vi "GraphSetting ScaleY (Wave2).vi"(6 "コマンド":T1, 8 "error in (no error)":errorcluster caption="エラー入力（エラーなし）", 9 "アクティブスケールY":u16, 10 "スケール(in)":T2, 11 "波形グラフ(Wave)ref(in)":refnum<vi>) -> (0 "error out":errorcluster caption="エラー出力", 2 "スケール(out)":T2)   [LabVIEW 2014]
uses:
  GraphSetting Scale.ctl
  TypeDef/GraphSetting DisplayFormatType.ctl
  TypeDef/GraphSetting Command.ctl
panel:
  # "スケールのスタイルとカラー"
  # "スケール係数"
  # "スケールのスタイルとカラー"
  # "スケールのスタイルとカラー"
  # "スケール係数"
  # "スケールのスタイルとカラー"
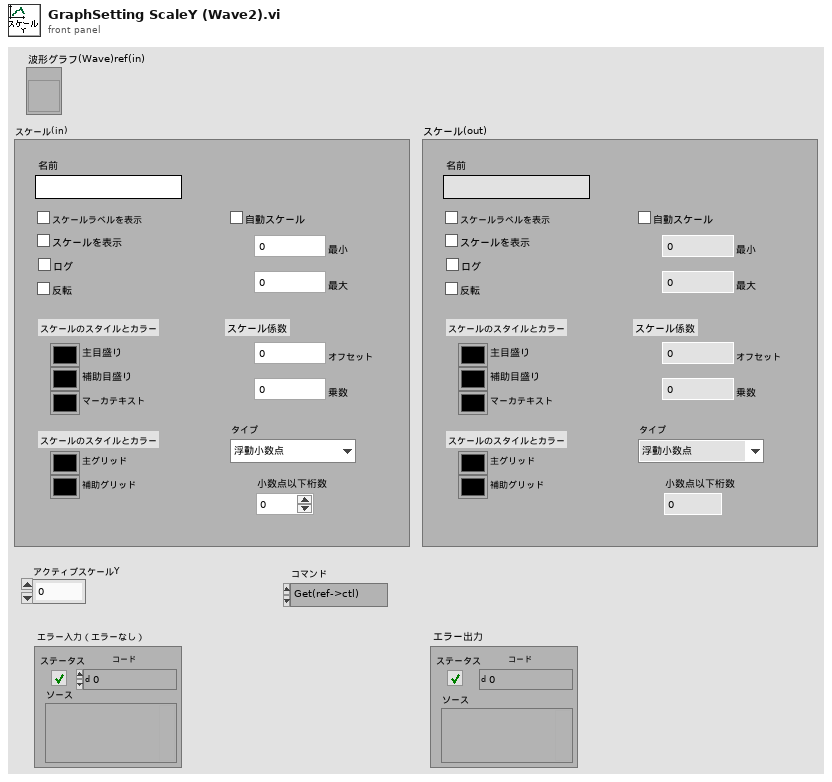
[diagram p1: front panel]
types:
  T1 = typedef "GraphSetting Command.ctl" = enum16{"Get(ref->ctl)", "Set(ctl->ref)"}
  T2 = typedef "GraphSetting Scale.ctl" = cluster{"名前":string, "スケールラベルを表示":bool, "スケールを表示":bool, "ログ":bool, "反転":bool, "自動スケール":bool, "最小":dbl, "最大":dbl, "オフセット":dbl, "乗数":dbl, "主目盛り":u32, "補助目盛り":u32, "マーカテキスト":u32, "主グリッド":u32, "補助グリッド":u32, "タイプ":T3, "小数点以下桁数":u8}
  T3 = typedef "GraphSetting DisplayFormatType.ctl" = enum8{"浮動小数点", "科学", "工学", "バイナリ", "８進数", "１６進数", "相対時間", "時間と日時", "SI"}
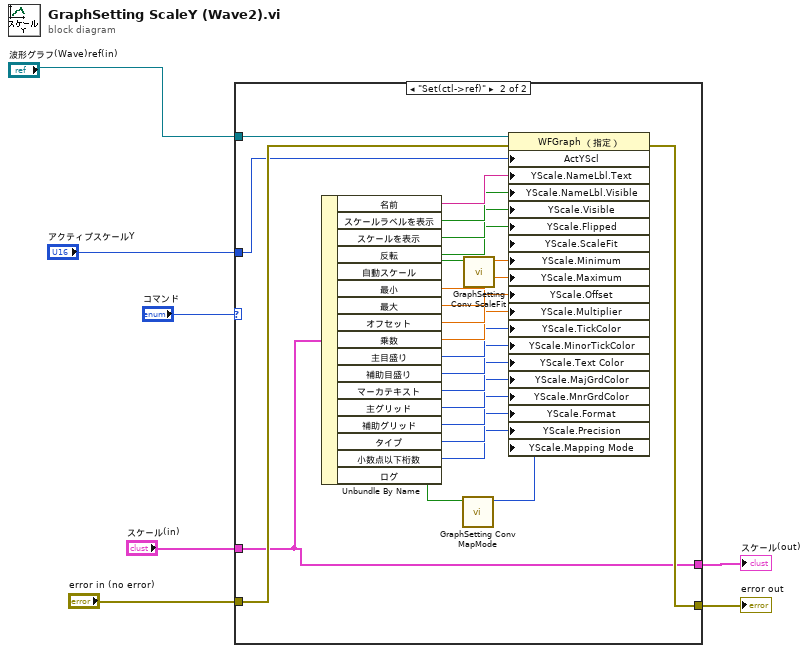
[diagram p0: block diagram]
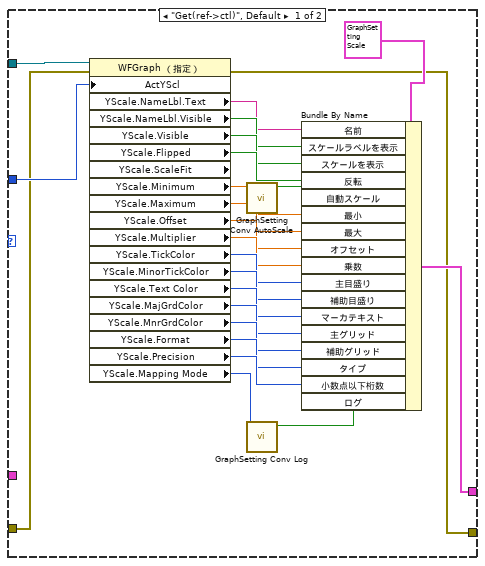
[diagram p2: hidden frame]
diagram:
  n1 = case shown="\"Set(ctl->ref)\"" "コマンド" {
    tunnel: "アクティブスケールY" -> [w16 w52]
    tunnel: "波形グラフ(Wave)ref(in)" -> [w15 w56]
    tunnel: [w14 w53] -> w6
    tunnel: [w13 w54] -> w4
    tunnel: "error in (no error)" -> [w12 w55]
    tunnel: "スケール(in)" -> [_ w53]
    frame "Get(ref->ctl)", Default {
      n2 = property class="WFGraph （指定）"(reference=w15, error in=w12, "ActYScl"=w16) -> (error out=w13:errorcluster, "YScale.NameLbl.Text"=w17:string, "YScale.NameLbl.Visible"=w18:bool, "YScale.Visible"=w19:bool, "YScale.Flipped"=w20:bool, "YScale.ScaleFit"=w11:u8, "YScale.Minimum"=w21:dbl, "YScale.Maximum"=w22:dbl, "YScale.Offset"=w23:dbl, "YScale.Multiplier"=w24:dbl, "YScale.TickColor"=w25:u32, "YScale.MinorTickColor"=w26:u32, "YScale.Text Color"=w27:u32, "YScale.MajGrdColor"=w28:u32, "YScale.MnrGrdColor"=w29:u32, "YScale.Format"=w30:u8, "YScale.Precision"=w31:u8, "YScale.Mapping Mode"=w9:u8)  [unwired: 1 out]
      n3 = call "GraphSetting Conv AutoScale.vi"("XScale.ScaleFit"=w11) -> ("自動スケール?"=w10:bool)  [unwired: 10 in]
      n4 = call "GraphSetting Conv Log.vi"("XScale.Mapping Mode"=w9) -> ("ログ?"=w8:bool)  [unwired: 10 in]
      n5 = Bundle By Name(cluster=T2 {"名前"="", "スケールラベルを表示"=FALSE, "スケールを表示"=FALSE, "ログ"=FALSE, "反転"=FALSE, "自動スケール"=FALSE, "最小"=0.0, "最大"=0.0, "オフセット"=0.0, "乗数"=0.0, "主目盛り"=0, "補助目盛り"=0, "マーカテキスト"=0, "主グリッド"=0, "補助グリッド"=0, "タイプ"=enum."浮動小数点", "小数点以下桁数"=0} ("スケール"), "名前"=w17, "スケールラベルを表示"=w18, "スケールを表示"=w19, "反転"=w20, "自動スケール"=w10, "最小"=w21, "最大"=w22, "オフセット"=w23, "乗数"=w24, "主目盛り"=w25, "補助目盛り"=w26, "マーカテキスト"=w27, "主グリッド"=w28, "補助グリッド"=w29, "タイプ"=w30, "小数点以下桁数"=w31, "ログ"=w8) -> (w14:T2)
    }
    frame "Set(ctl->ref)" {
      n6 = Unbundle By Name(w53) -> ("名前"=w51:string, "スケールラベルを表示"=w50:bool, "スケールを表示"=w49:bool, "反転"=w48:bool, "自動スケール"=w36:bool, "最小"=w47:dbl, "最大"=w46:dbl, "オフセット"=w45:dbl, "乗数"=w44:dbl, "主目盛り"=w43:u32, "補助目盛り"=w42:u32, "マーカテキスト"=w41:u32, "主グリッド"=w40:u32, "補助グリッド"=w39:u32, "タイプ"=w38:T3, "小数点以下桁数"=w37:u8, "ログ"=w34:bool)
      n7 = call "GraphSetting Conv MapMode.vi"("ログ"=w34) -> ("Xスケール.マッピングモード"=w33:u8)  [unwired: 10 in]
      n8 = call "GraphSetting Conv ScaleFit.vi"("自動スケール?"=w36) -> ("Xスケール.スケールフィット"=w35:u8)  [unwired: 10 in]
      n9 = property class="WFGraph （指定）"(reference=w56, error in=w55, "ActYScl"=w52, "YScale.NameLbl.Text"=w51, "YScale.NameLbl.Visible"=w50, "YScale.Visible"=w49, "YScale.Flipped"=w48, "YScale.ScaleFit"=w35, "YScale.Minimum"=w47, "YScale.Maximum"=w46, "YScale.Offset"=w45, "YScale.Multiplier"=w44, "YScale.TickColor"=w43, "YScale.MinorTickColor"=w42, "YScale.Text Color"=w41, "YScale.MajGrdColor"=w40, "YScale.MnrGrdColor"=w39, "YScale.Format"=w38, "YScale.Precision"=w37, "YScale.Mapping Mode"=w33) -> (error out=w54:errorcluster)  [unwired: 1 out]
    }
  }
  "スケール(out)" <- w6
  "error out" <- w4
